vi "CheckSum19073.vi"(11 "Array":u8[](array[numeric])) -> (3 "data string":string)   [LabVIEW 2016]
doc: "Input : Array of bytes convert from string (except chechsum)\nout put : checksum as string"
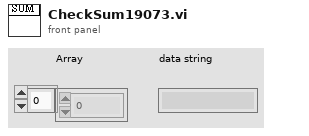
[diagram p1: front panel]
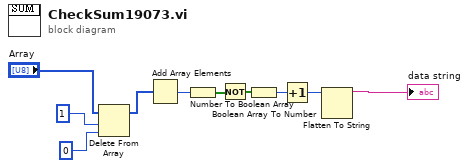
[diagram p0: block diagram]
diagram:
  n1 = Delete From Array(array="Array", length=1, index=0) -> (array with subset deleted=w10:u8[])  [unwired: 1 out]
  n2 = Add Array Elements(numeric array=w10) -> (sum=w1:u8)
  n3 = Number To Boolean Array(number=w1) -> (Boolean array=w2:bool[])
  n4 = Not(x=w2) -> (.not. x?=w3:bool[])
  n5 = Boolean Array To Number(Boolean array=w3) -> (number=w4:u8)
  n6 = Increment(x=w4) -> (x+1=w5:u8)
  n7 = Flatten To String(anything=w5) -> (data string=→"data string":string)  [unwired: 3 in, 2 out]
